vi "VLC - Play_Discrete_fps.vi"(5 "Media Source":string="rtsp://admin:admin@192.168.1.108/cam/realmonitor?channel=1&subtype=0", 7 "Script":string=" network-caching=200", 11 "error in (no error)":errorcluster) -> (15 "error out":errorcluster)   [LabVIEW 2016]
uses:
  System.Windows.Forms
panel:
  in  "FramePerSec":i32=3 max=10
  in  "stop":bool
  out "Slide":u8(slide) scale=0.0..100.0
  out "timed out?":bool
  in  "Image":T1(plugin-control)
  out "LoopTime":u32
  in  "PictureBox":refnum<k24>(container)
  # "rtsp://admin:admin@192.168.1.108/cam/realmonitor?channel=1&subtype=1"
  # "rtsp://admin:gamma2018@84.253.163.35:554/cam/realmonitor?channel=1&subtype=1"
  # "the target computer for the application must have the .NET Framework 4.0 installed."
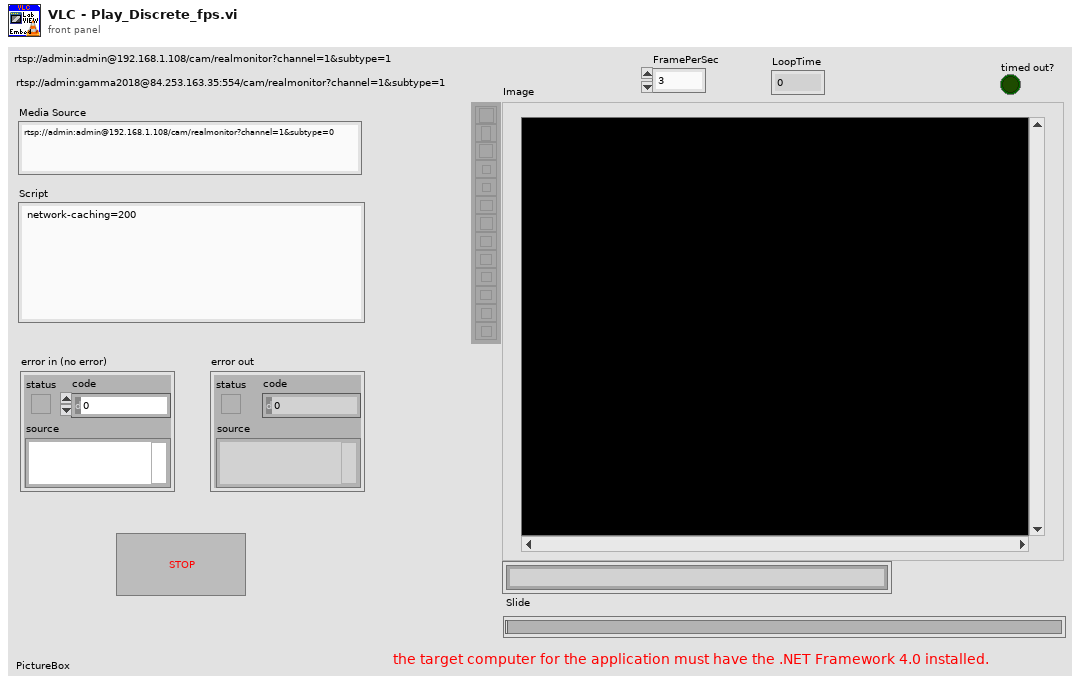
[diagram p1: front panel]
types:
  T1 = typedef "IMAQ Image.ctl" = refnum<image>
  T2 = typedef "Image Type" = u32
  T3 = typedef "VLC-IP.ctl" = cluster{"path of VLC":path, "VLC media player pointer":i32, "VLC Istance pointer":i32, "p_mi":i32}
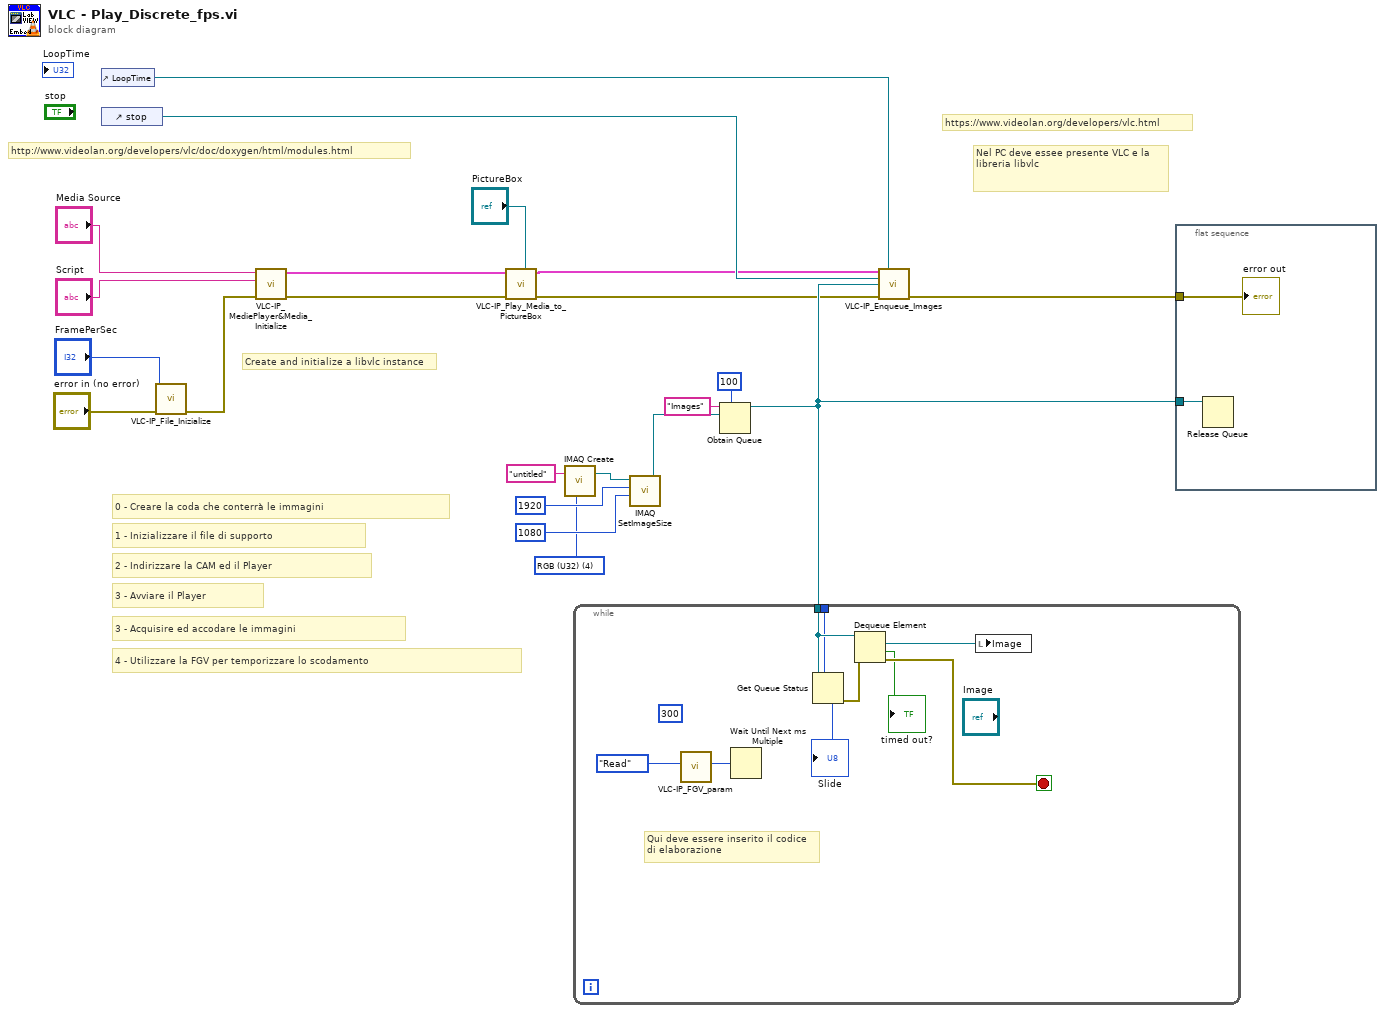
[diagram p0: block diagram]
diagram:
  w2 = T2 4 items=["Grayscale (U8)", "Grayscale (I16)", "Grayscale (SGL)", "Complex (CSG)", "RGB (U32)", "HSL (U32)", "RGB (U64)", "Grayscale (U16)"] ("Image Type")
  # "0 - Creare la coda che conterrà le immagini"
  # "4 - Utilizzare la FGV per temporizzare lo scodamento"
  # "3 - Acquisire ed accodare le immagini"
  # "3 - Avviare il Player"
  # "2 - Indirizzare la CAM ed il Player"
  # "1 - Inizializzare il file di supporto"
  # "https://www.videolan.org/developers/vlc.html"
  # "Nel PC deve essee presente VLC e la \nlibreria libvlc"
  # "Create and initialize a libvlc instance"
  # "http://www.videolan.org/developers/vlc/doc/doxygen/html/modules.html"
  n1 = control-ref of="LoopTime"() -> (w10:refnum<vi>)
  n2 = control-ref of="stop"() -> (w9:refnum<vi>)
  n3 = call "VLC-IP_File_Inizialize.vi"("error in"="error in (no error)", "FramePerSec"="FramePerSec") -> ("error out"=w15:errorcluster)  [unwired: 7 in, 2 out]
  n4 = call "VLC-IP_MediePlayer&Media_Initialize.vi"("error in (no error)"=w15, "Script"="Script", "Media Source"="Media Source") -> ("error out"=w22:errorcluster, "VLC-IP"=w13:T3)  [unwired: 7 in]
  n5 = call "VLC-IP_Play_Media_to_PictureBox.vi"(".NET PictureBox"="PictureBox", "error in (no error)"=w22, "VLC-IP"=w13) -> ("error out"=w7:errorcluster, "VLC-IP out"=w8:T3)  [unwired: 7 in]
  n6 = call "IMAQ Create"("Image Name"="untitled", "Image Type"=w2) -> ("New Image"=w3:T1)  [unwired: 3 in, 1 out]
  n7 = call "IMAQ SetImageSize"("Y Resolution"=1080 ("X Resolution"), "X Resolution"=1920, "Image"=w3) -> ("Image Out"=w4:T1)  [unwired: 2 in, 1 out]
  n8 = Obtain Queue(max queue size (-1, unlimited)=100, name (unnamed)="Images", element data type=w4) -> (queue out=w11:refnum<queue>)  [unwired: 2 in, 2 out]
  n9 = while {
    tunnel: w11 -> [w28]
    tunnel: [w25] -> _
    stop <- w31 stop-if-true
    (unwired) 300
    # "Qui deve essere inserito il codice\ndi elaborazione"
    n10 = call "VLC-IP_FGV_param.vi"("Mode"=enum16{"Read", "Write"}."Read") -> ("SamplingTime_out"=w23:i32)  [unwired: 9 in, 1 out]
    n11 = Wait Until Next ms Multiple(millisecond multiple=w23) -> ()  [unwired: 1 out]
    n12 = Get Queue Status(queue=w28) -> (max queue size=w25:i32, error out=w27:errorcluster, # elements in queue=→"Slide":i32)  [unwired: 2 in, 5 out]
    n13 = Dequeue Element(queue=w28, error in (no error)=w27) -> (element=w30:T1, timed out?=→"timed out?":bool, error out=w31:errorcluster)  [unwired: 1 in, 1 out]
    n14 = local write "Image"(w30) -> ()
  }
  n15 = call "VLC-IP_Enqueue_Images.vi"("VLC-IP"=w8, "dTime"=w10, "Stop in"=w9, "queue in"=w11, "error in (no error)"=w7) -> ("error out"=w19:errorcluster)  [unwired: 10 in]
  n16 = flat-sequence {
    tunnel: w19 -> [w33]
    tunnel: w11 -> [w32]
    frame #0 {
      n17 = Release Queue(queue=w32) -> ()  [unwired: 2 in, 3 out]
      "error out" <- w33
    }
  }
